vi "FdxCmdMonQueueReadCvi.vi"(6 "MaxReadBytes":u32=65535, 7 "ReadQualifier":u32(ring) items=["FDX_MON_READ_FULL", "FDX_MON_READ_HEADER", "FDX_MON_READ_DATA"], 8 "error in":errorcluster, 9 "EntryCount":u32=1, 10 "QueueId":u32, 11 "InstrumentHandle_port":u32) -> (0 "error out":errorcluster, 1 "QueueReadOut":T1, 2 "QueueIdOut":u32, 3 "InstrumentHandle_port":u32)   [LabVIEW 2020, in "AIM664LV.lvlib"]
doc: "This function is used to read Entries of a chronological capturing queue to a provided buffer. For this read function only the number of Entries to be read is specified. The reading start position is administrated internal to the target. The start position can by identified and modified by the functions AiFdxCmdMonQueueTell(...) and AiFdxCmdMonQueueSeek(...). Additional processing, for accessing the Frame Header data must be done via AiFdxProcessMonQueue function.\nNote: Data, read via AiFdxCmdMonQueueRead, can be directly used for Replay via the AiFdxCmdTxQueueWrite function, if the corresponding Transmit Port has been configured for Replay."
uses:
  AIM664LV.lvlib
  AFDX_LibraryAdmin/FdxGlobalDllPath.vi
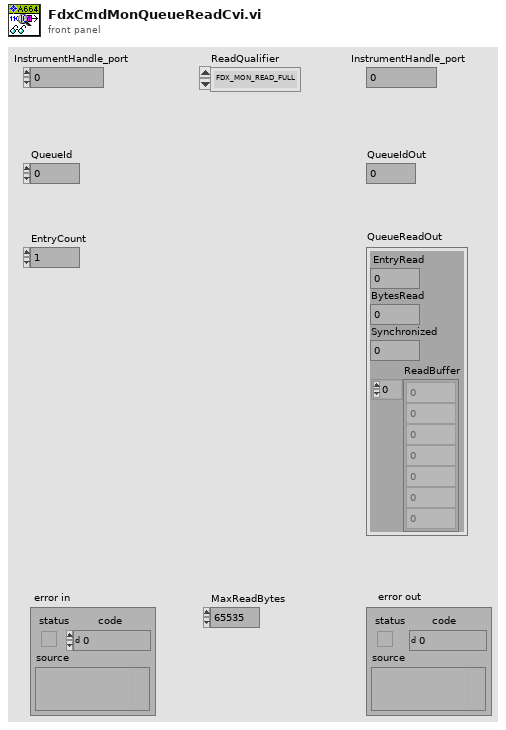
[diagram p1: front panel]
types:
  T1 = cluster{"EntryRead":u32, "BytesRead":u32, "Synchronized":u32, "ReadBuffer":u8[]}
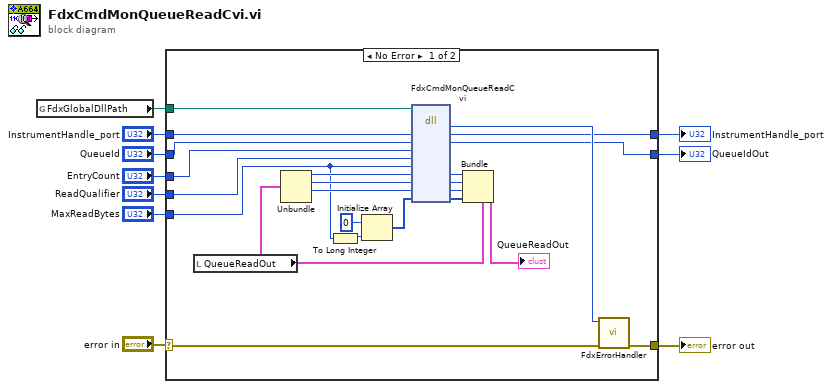
[diagram p0: block diagram]
diagram:
  n1 = global read "FdxGlobalDllPath.vi" "FdxGlobalDllPath"() -> (w8:path)
  n2 = case shown="No Error" "error in" {
    selector: "error in" -> [w32 w36]
    tunnel: [w33 w36] -> w10
    tunnel: w8 -> [w18 _]
    tunnel: "InstrumentHandle_port" -> [w17 w35]
    tunnel: [w16 w35] -> w6
    tunnel: "QueueId" -> [w15 w34]
    tunnel: "EntryCount" -> [w14 _]
    tunnel: "ReadQualifier" -> [w13 _]
    tunnel: "MaxReadBytes" -> [w12 _]
    tunnel: [w11 w34] -> w1
    frame No Error {
      n3 = local read "QueueReadOut"() -> (w19:T1)
      n4 = Unbundle(w19) -> ("EntryRead"=w22:u32, "BytesRead"=w21:u32, "Synchronized"=w20:u32)  [unwired: 1 out]
      n5 = To Long Integer(number=w12) -> (32bit integer=w23:i32)
      n6 = Initialize Array(u8 0 ("element"), w23) -> (w30:u8[])
      n7 = dll-call lib="aim_fdx.19.dll" fn="FdxCmdMonQueueReadCvi"(path in=w18, "InstrumentHandle"=w17, "QueueId"=w15, "EntryCount"=w14, "ReadQualifier"=w13, "MaxReadBytes"=w12, "EntryRead"=w22, "BytesRead"=w21, "Synchronized"=w20, "ReadBuffer"=w30) -> ("status"=w31:i32, "InstrumentHandle"=w16:u32, "QueueId"=w11:u32, "EntryRead"=w28:u32, "BytesRead"=w27:u32, "Synchronized"=w26:u32, "ReadBuffer"=w25:u8[])  [unwired: 5 in, 2 out]
      n8 = Bundle(cluster=w19, "EntryRead"=w28, "BytesRead"=w27, "Synchronized"=w26, "ReadBuffer"=w25) -> (→"QueueReadOut":T1)
      n9 = call "FdxErrorHandler.vi"("error in"=w32, "AIM Error"=w31) -> ("error out"=w33:errorcluster)  [unwired: 9 in]
    }
    frame Error {
    }
  }
  "error out" <- w10
  "InstrumentHandle_port" <- w6
  "QueueIdOut" <- w1
